vi "GameStateMachine.vi"(0 "Input Playfield":bool[][](array[boolean]), 5 "Tile Info Input":T1, 9 "Input Reset":bool, 11 "Enum":T2) -> (4 "Output Playfield":bool[][](array[boolean]), 6 "Tile Info Output":T1, 10 "Game over":bool)   [LabVIEW 2026]
doc: "VI used for storing, tracking and controlling the state of the game."
uses:
  01_Typen/GameCommandTypeDef.ctl
  GameTetrominoInformationTypeDef.ctl
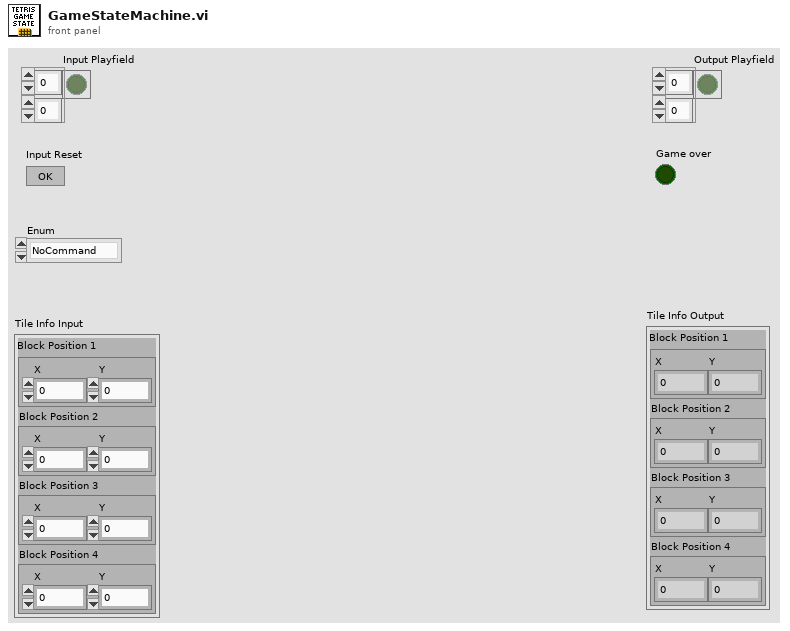
[diagram p1: front panel]
types:
  T1 = typedef "GameTetrominoInformationTypeDef.ctl" = cluster{"Block Position 1":cluster{"X":i32, "Y":i32}, "Block Position 2":cluster{"X":i32, "Y":i32}, "Block Position 3":cluster{"X":i32, "Y":i32}, "Block Position 4":cluster{"X":i32, "Y":i32}}
  T2 = typedef "GameCommandTypeDef.ctl" = enum16{"NoCommand", "Rotate", "MoveLeft", "MoveRight"}
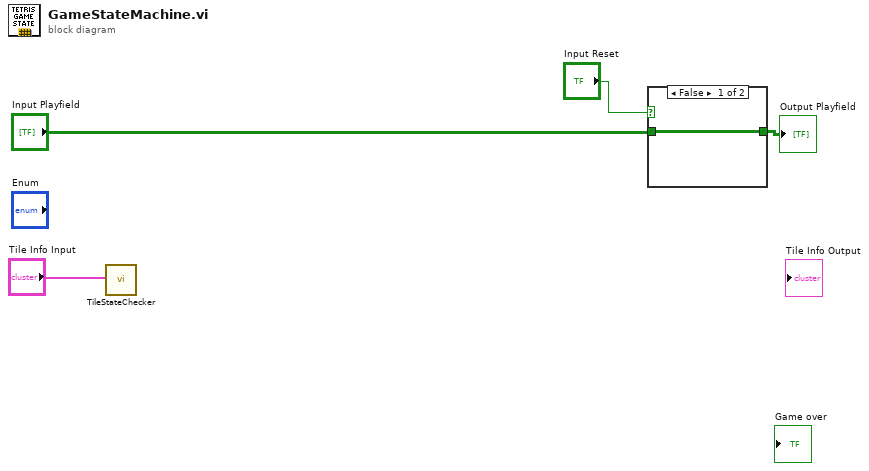
[diagram p0: block diagram]
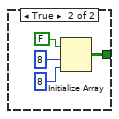
[diagram p2: hidden frame]
diagram:
  n1 = call "TileStateChecker.vi"("Tile Info"="Tile Info Input") -> ()  [unwired: 8 in, 1 out]
  n2 = case shown="False" "Input Reset" {
    tunnel: "Input Playfield" -> [w5 _]
    tunnel: [w5 w6] -> w3
    frame False {
    }
    frame True {
      n3 = Initialize Array(FALSE, 8 ("dimension size"), 8 ("dimension size")) -> (w6:bool[][])
    }
  }
  "Output Playfield" <- w3
